vi "getTestCaseInstanceName.vi"(11 "TestCase in":refnum<class "TestCase.lvclass">) -> (2 "Test Case Instance Name":string, 3 "TestCase out":refnum<class "TestCase.lvclass">)   [LabVIEW 2013, in "TestCase.lvclass"]
doc: "Gets the name for this instance of the test case. This is the name that will appear in the user interface."
uses:
  TestCase.lvclass
  TestCase.lvclass/TestCase.ctl
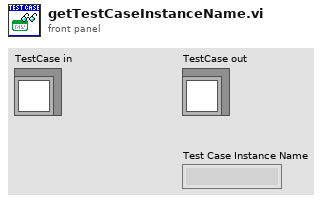
[diagram p1: front panel]
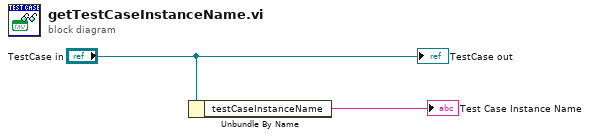
[diagram p0: block diagram]
diagram:
  n1 = Unbundle By Name("TestCase in") -> ("testCaseInstanceName"=→"Test Case Instance Name":string)
  "TestCase out" <- "TestCase in"
